vi "SDO download (U16).vi"(4 "Value":u16, 5 "Wait?":bool, 6 "error in (no error)":errorcluster, 7 "Multiplexor":T1 {"Sub-index" format="%02x"; "Index" format="%04x"}, 8 "Node ID":u8, 9 "CANopen in":refnum<class "CANopen.lvclass">) -> (0 "error out":errorcluster, 3 "CANopen out":refnum<class "CANopen.lvclass">)   [LabVIEW 2017, in "canopen.lvlib" / "CANopen.lvclass"]
doc: "Writes a value in the open dictionary of a CANopen node."
uses:
  CANopen.lvclass
  Multiplexor.ctl
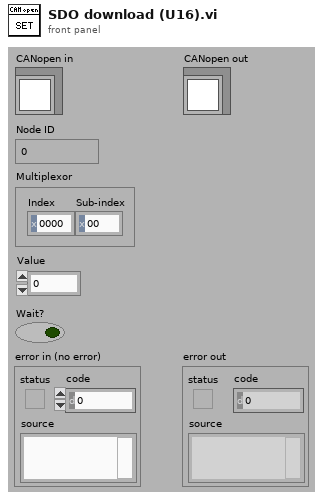
[diagram p1: front panel]
types:
  T1 = typedef "canopen.lvlib/CANopen.lvclass/Multiplexor.ctl" = cluster{"Index":u16, "Sub-index":u8}
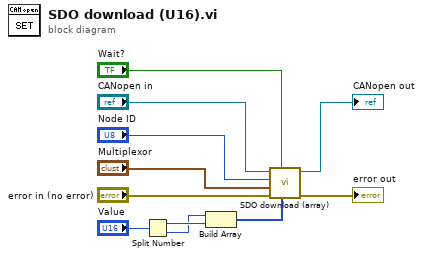
[diagram p0: block diagram]
diagram:
  n1 = Split Number(x="Value") -> (hi(x)=w4:u8, lo(x)=w3:u8)
  n2 = Build Array(w3, w4) -> (w5:u8[])
  n3 = call "SDO download (array).vi"("Value"=w5, "Wait?"="Wait?", "error in (no error)"="error in (no error)", "Multiplexor"="Multiplexor", "Node ID"="Node ID", "CANopen in"="CANopen in") -> ("error out"=→"error out":errorcluster, "CANopen out"=→"CANopen out":refnum<class "CANopen.lvclass">)  [unwired: 2 out]
